vi "Get From Type Descriptor Map.vi"(8 "error in (no error)":errorcluster, 10 "Type Name":string, 11 "TwinCAT ADS in":refnum<class "TwinCAT ADS.lvclass">) -> (0 "error out":errorcluster, 1 "Found?":bool, 2 "Type Descriptor":i16[](array[numeric]), 3 "TwinCAT ADS out":refnum<class "TwinCAT ADS.lvclass">)   [LabVIEW 2018, in "TwinCAT ADS.lvclass"]
uses:
  TwinCAT ADS.lvclass
  TwinCAT ADS.lvclass/TwinCAT ADS.ctl
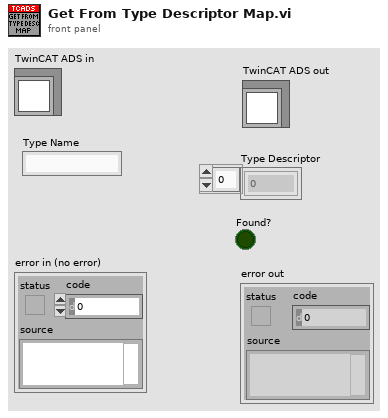
[diagram p1: front panel]
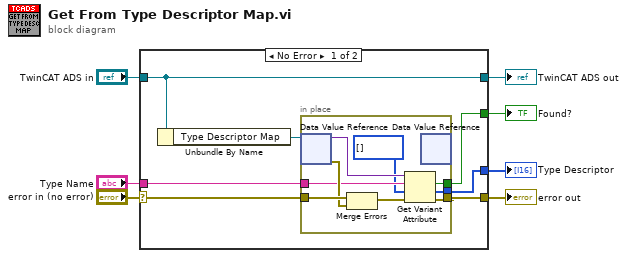
[diagram p0: block diagram]
diagram:
  n1 = case shown="No Error" "error in (no error)" {
    selector: "error in (no error)" -> [w9 w25]
    tunnel: [w12 w25] -> w6
    tunnel: [w14 w24] -> w4
    tunnel: "TwinCAT ADS in" -> [w14 w24]
    tunnel: "Type Name" -> [w8 _]
    tunnel: [w11 _] -> w1
    tunnel: [w10 _] -> w2
    frame No Error {
      n2 = Unbundle By Name(w14) -> ("Type Descriptor Map"=w13:refnum<data-value>)
      n3 = in-place {
        in-place-border: w8 -> [w19]
        in-place-border: w9 -> [w21]
        in-place-border: [w17] -> w11
        in-place-border: [w16] -> w10
        in-place-border: [w15] -> w12
        n4 = in-place-dvr #1(w13) -> (w23:variant, w20:errorcluster)
        n5 = Merge Errors(w21, w20) -> (w22:errorcluster)
        n6 = Get Variant Attribute(Variant=w23, name=w19, default value (empty Variant)=i16[] [] ("Type Descriptor"), error in=w22) -> (found=w17:bool, value=w16:i16[], error out=w15:errorcluster)  [unwired: 1 out]
        n7 = in-place-dvr #1() -> ()  [unwired: 1 in, 2 out]
      }
    }
    frame Error {
    }
  }
  "error out" <- w6
  "TwinCAT ADS out" <- w4
  "Type Descriptor" <- w2
  "Found?" <- w1
